vi "CR-导丝颗粒物检测3.vi"(8 "error in (no error)":errorcluster caption="错误输入（无错误）", 11 "名称或相对路径":string="Template Program") -> (0 "error in (no error) 2":errorcluster caption="错误输入（无错误）")   [LabVIEW 2017]
uses:
  Global System.vi
  <vilib>/Utility/xml.llb/Write to XML File(string).vi
  Picture/SaveButtom.ctl
panel:
  in  "获取图像":bool
  in  "ROI获取":bool
  in  "创建模板":bool
  in  "保存图像":bool
  out "添加的路径":path
  in  "刷新":bool
  in  "测试按钮":bool
  in  "保存按钮":bool
  in  "Main":enum32{"主参数", "模板匹配参数 ", "测试效果"}(tab)
  in  "导丝颗粒物检测3基础参数":T1={"IsNorImage"=TRUE, "Exposure Values"=100289, "ImagePath"=path "C:/Users/hedongpo/Desktop/514-hdp/Alignment Assemble System/Test Picture/B/3.bmp"} caption="参数界面" {"Exposure Values" scale=0.0..200000.0}
  in  "导丝颗粒物检测3参数":T3={"Rectangle"={"Left"=0, "Top"=0, "Right"=0, "Bottom"=0, "Rotation"=0.0}, "Threshold Limits (Threshold 1)"={"Lower value"=6.0, "Upper value"=245.0}, "Keep/Remove Particles "=FALSE, "Connectivity 4/8 (8) "=TRUE, "Selection Values (Particle Filter 1)"=[{"Measurement Parameter"=35, "Range Lower Value"=80.0, "Range Upper Value"=16332.0, "Range"=FALSE, "Measurement Type"=FALSE}], "Corner Options (Feature Detection 1)"={"Detector type"=enum."Harris Corner", "Kernel size"=7, "Min Corner Point Strength"=32.0}, "Pyramid level (Feature Detection 1)"=3, "Method "=2, "Look For"=0, "Method 2"=2, "ROI Descriptor (Clamp (Rake) 1)"={"Global Rectangle"=[162, 394, 420, 1807], "Contours"=[{"ID"=enum."External", "Type"=12, "Coordinates"=[162, 394, 420, 1807, 0]}]}} {"Method" items=["clustering", "entropy", "metric", "moments", "inter-class variance"]; "Look For" items=["Bright Objects", "Dark Objects"]; "Method 2" items=["clustering", "entropy", "metric", "moments", "inter-class variance"]; "ROI Descriptor (Clamp (Rake) 1)"."Contours"."Type" items=["No Selection", "Point", "Line", "Rectangle", "Oval", "Polygon", "Freehand Region", "Annulus", "Unused2", "Unused3", "Broken Line", "Freehand Line", "Rotated Rectangle"]; "Selection Values (Particle Filter 1)"."Measurement Parameter" items=["Center of Mass X", "Center of Mass Y", "First Pixel X", "First Pixel Y", "Bounding Rect Left", "Bounding Rect Top", "Bounding Rect Right", "Bounding Rect Bottom", "Max Feret Diameter Start X", "Max Feret Diameter Start Y", "Max Feret Diameter End X", "Max Feret Diameter End Y", "Max Horiz. Segment Length Left", "Max Horiz. Segment Length Right", "Max Horiz. Segment Length Row", "-", "Bounding Rect Width", "Bounding Rect Height", "Bounding Rect Diagonal", "Perimeter", "Convex Hull Perimeter", "Holes' Perimeter", "Max Feret Diameter", "Equivalent Ellipse Major Axis", "Equivalent Ellipse Minor Axis", "Equivalent Ellipse Minor Axis (Feret)", "Equivalent Rect Long Side", "Equivalent Rect Short Side", "Equivalent Rect Diagonal", "Equivalent Rect Short Side (Feret)", "Average Horiz. Segment Length", "Average Vert. Segment Length", "Hydraulic Radius", "Waddel Disk Diameter", "-", "Area", "Holes' Area", "Particle & Holes' Area", "Convex Hull Area", "Image Area", "-", "Number of Holes", "Number of Horiz. Segments", "Number of Vert. Segments", "-", "Orientation", "Max Feret Diameter Orientation", "-", "% Area/Image Area", "% Area/(Particle & Holes' Area)", "Ratio of Equivalent Ellipse Axes", "Ratio of Equivalent Rect Sides", "-", "Elongation Factor", "Compactness Factor", "Heywood Circularity Factor", "Type Factor", "-", "Sum X", "Sum Y", "Sum XX", "Sum XY", "Sum YY", "Sum XXX", "Sum XXY", "Sum XYY", "Sum YYY", "-", "Moment of Inertia XX", "Moment of Inertia XY", "Moment of Inertia YY", "Moment of Inertia XXX", "Moment of Inertia XXY", "Moment of Inertia XYY", "Moment of Inertia YYY", "Norm. Moment of Inertia XX", "Norm. Moment of Inertia XY", "Norm. Moment of Inertia YY", "Norm. Moment of Inertia XXX", "Norm. Moment of Inertia XXY", "Norm. Moment of Inertia XYY", "Norm. Moment of Inertia YYY", "Hu Moment 1", "Hu Moment 2", "Hu Moment 3", "Hu Moment 4", "Hu Moment 5", "Hu Moment 6", "Hu Moment 7"]; "Rectangle"."Rotation" min=-90.0 max=90.0 step=1.0 format="%.2f"; "Rectangle"."Left" scale=0.0..1024.0; "Rectangle"."Right" scale=0.0..1024.0}
  out "颗粒物有无显示":bool
  out "Number of Features Found":i32
  in  "颗粒物个数阈值":i32
  in  "Feature Points Strength":string[][](table)
  out "原始图像":T4(plugin-control)
  out "路径输出":path
  in  "Vision Paramter Save Buttom":T5
  out "system time":string
  in  "取消按钮":bool
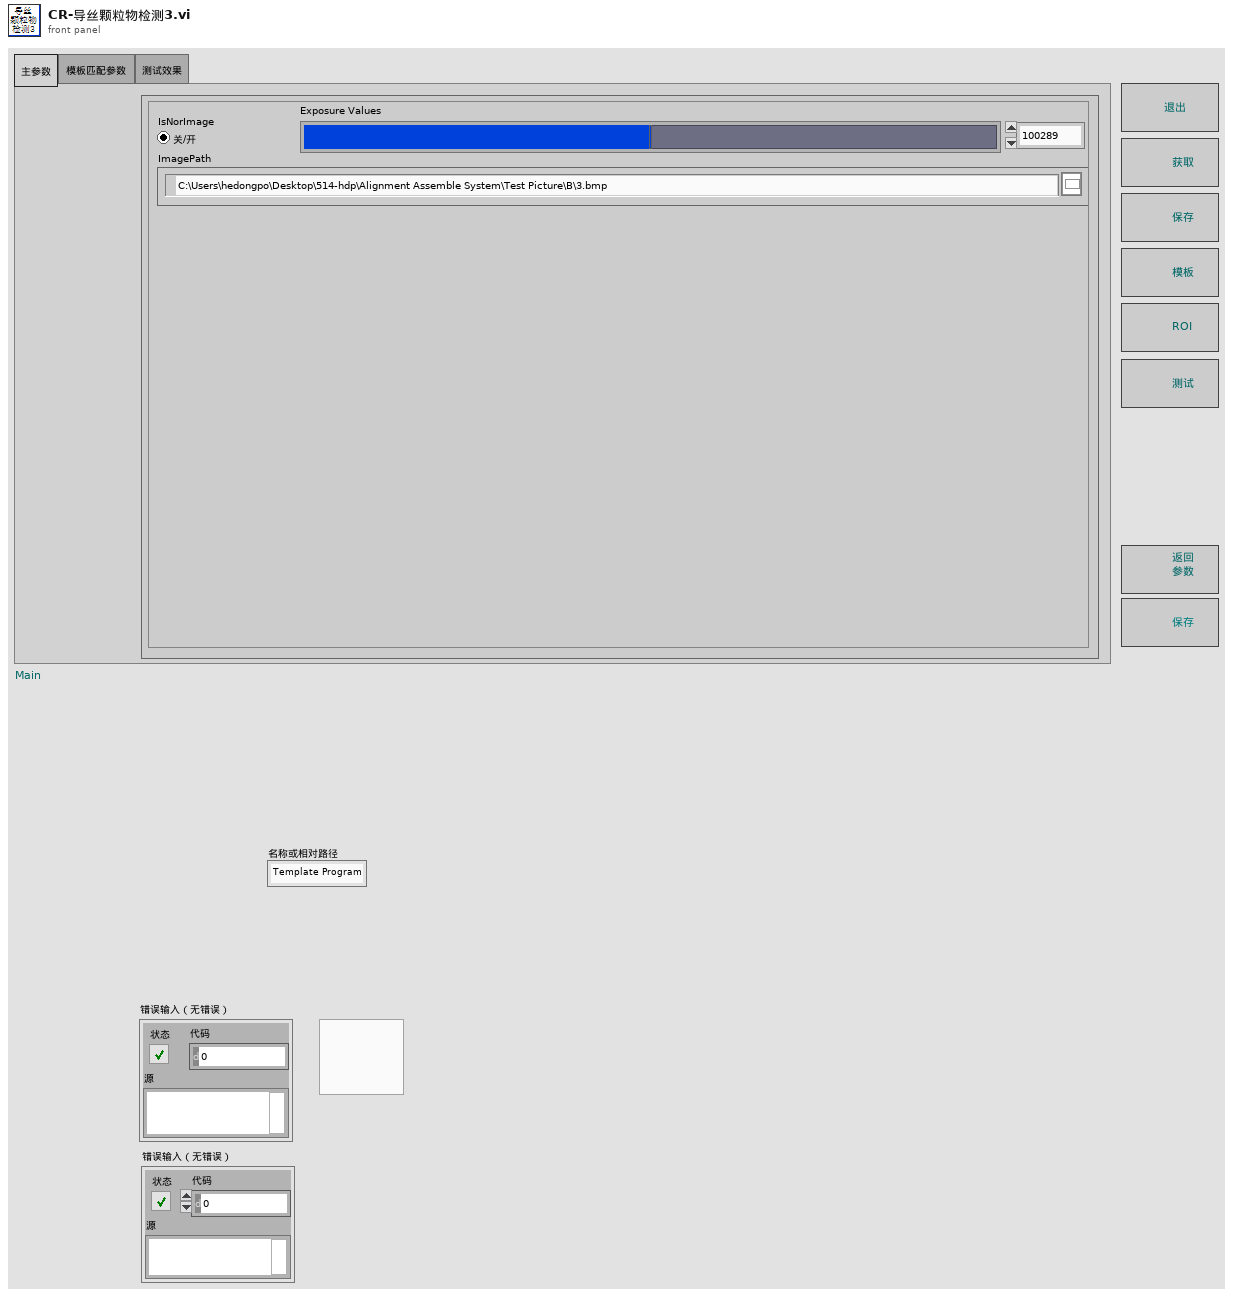
[diagram p1: front panel]
types:
  T1 = cluster{"IsNorImage":bool, "Exposure Values":u32, "ImagePath":path}
  T2 = typedef "IMAQ Rectangle" = cluster{"Left":i32, "Top":i32, "Right":i32, "Bottom":i32, "Rotation":dbl}
  T3 = cluster{"Rectangle":T2, "Threshold Limits (Threshold 1)":cluster{"Lower value":sgl, "Upper value":sgl}, "Keep/Remove Particles ":bool, "Connectivity 4/8 (8) ":bool, "Selection Values (Particle Filter 1)":cluster{"Measurement Parameter":i32, "Range Lower Value":dbl, "Range Upper Value":dbl, "Range":bool, "Measurement Type":bool}[], "Corner Options (Feature Detection 1)":cluster{"Detector type":enum32{"Harris Corner", "Shi-Tomasi Corner"}, "Kernel size":i32, "Min Corner Point Strength":dbl}, "Pyramid level (Feature Detection 1)":u32, "Method ":i32, "Look For":u32, "Method 2":i32, "ROI Descriptor (Clamp (Rake) 1)":cluster{"Global Rectangle":i32[], "Contours":cluster{"ID":enum32{"External", "Internal"}, "Type":u32, "Coordinates":i32[]}[]}}
  T4 = typedef "IMAQ Image.ctl" = refnum<image>
  T5 = typedef "SaveButtom.ctl" = bool
  T6 = cluster{"index":i32, "this vi":refnum<vi>, "error out":errorcluster}
  T7 = cluster{"master data":string, "priority":u16, "secondary data":string[]}
  T8 = cluster{"case name":string[], "queue array":refnum<queue>[]}
  T9 = cluster{"Global Rectangle":i32[], "Contours":cluster{"Contour Type":u32, "ROI Type":u32, "Points":i32[]}[]}
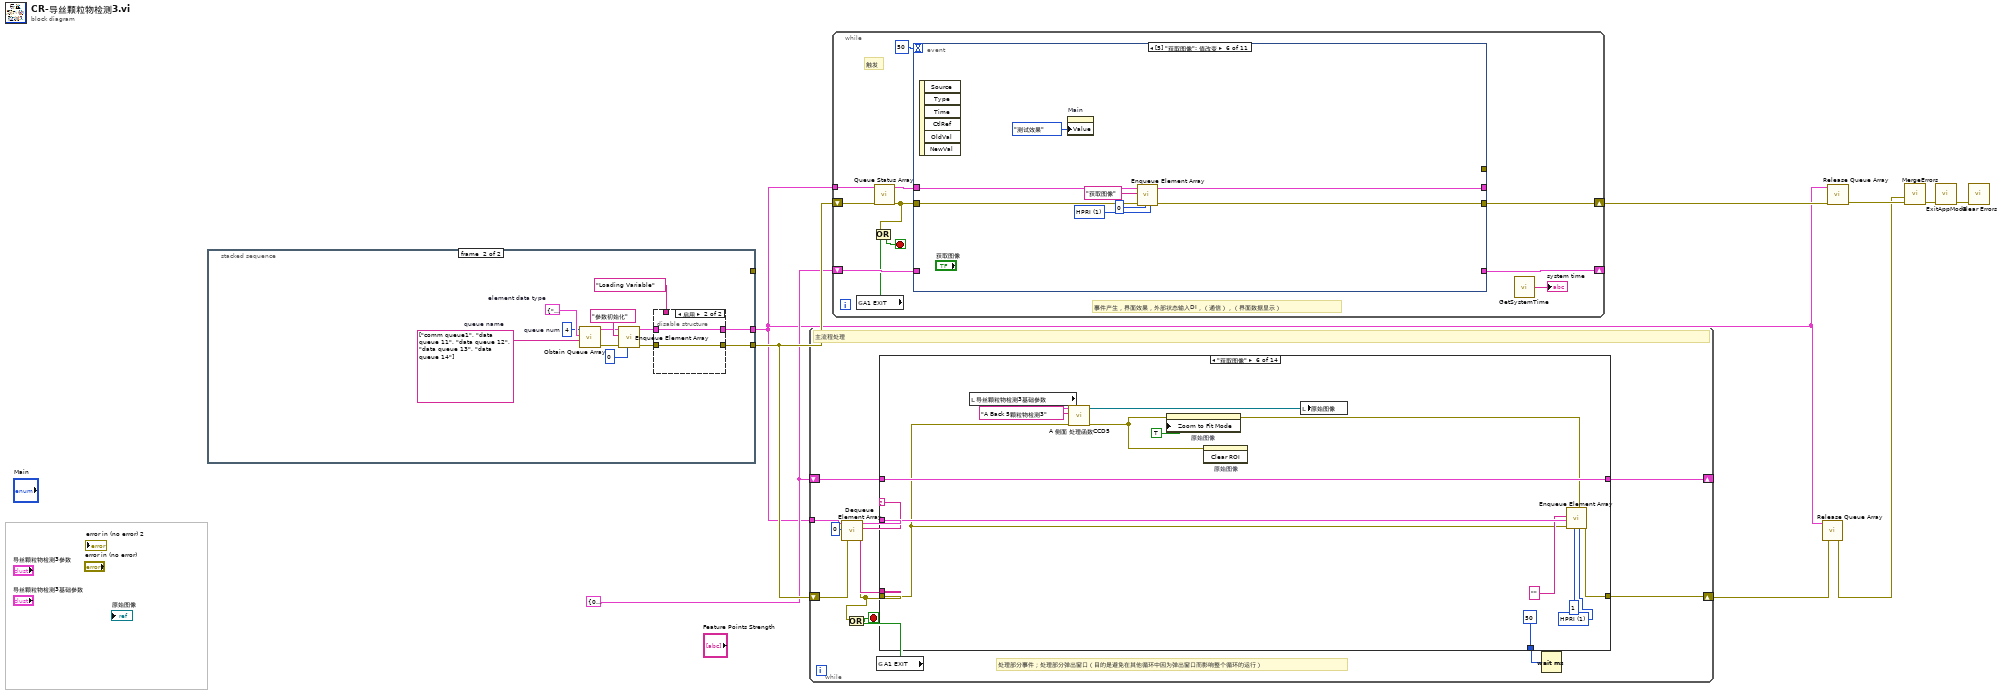
[diagram p0: block diagram]
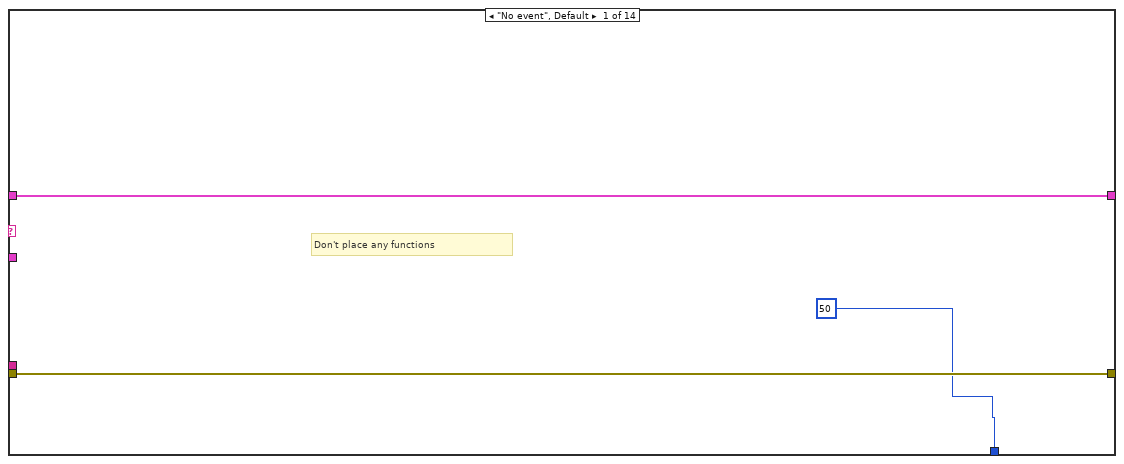
[diagram p2: hidden frame]
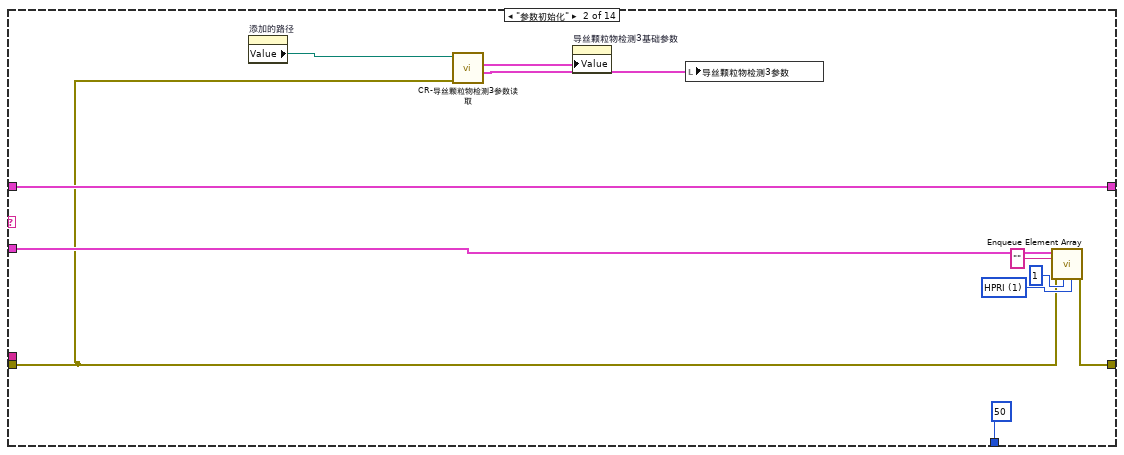
[diagram p3: hidden frame]
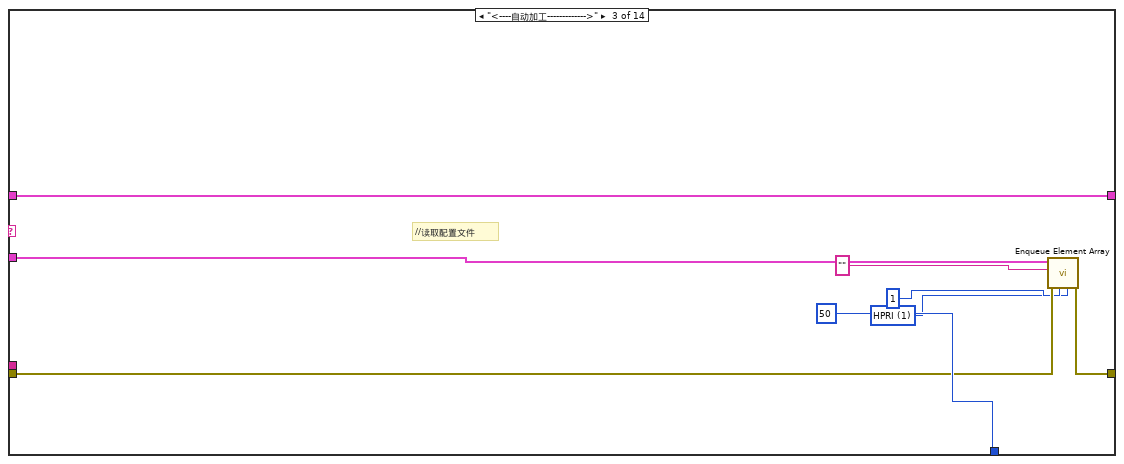
[diagram p4: hidden frame]
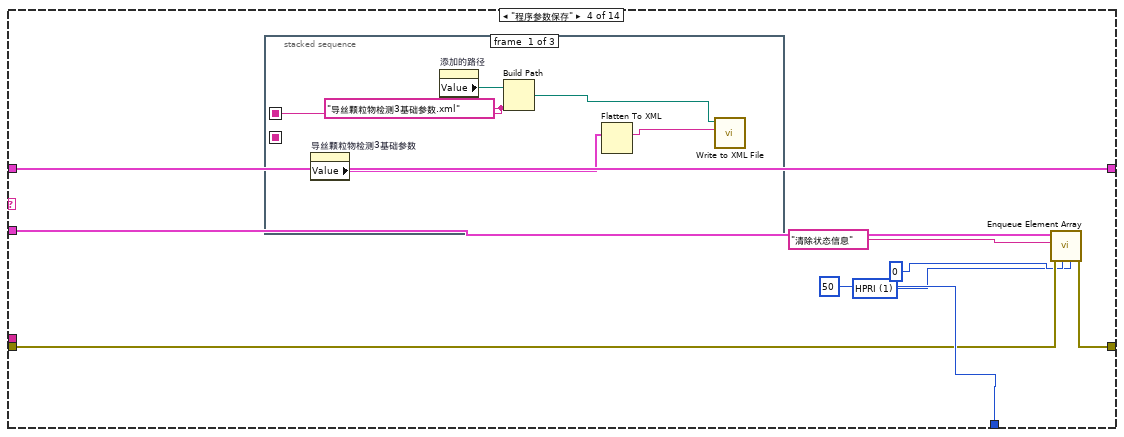
[diagram p5: hidden frame]
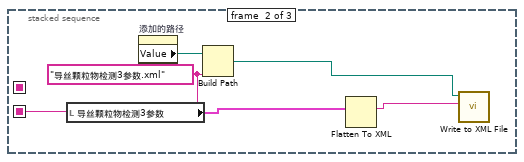
[diagram p6: hidden frame]
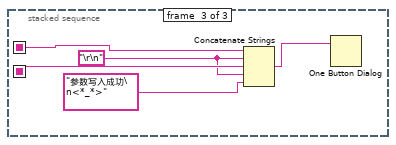
[diagram p7: hidden frame]
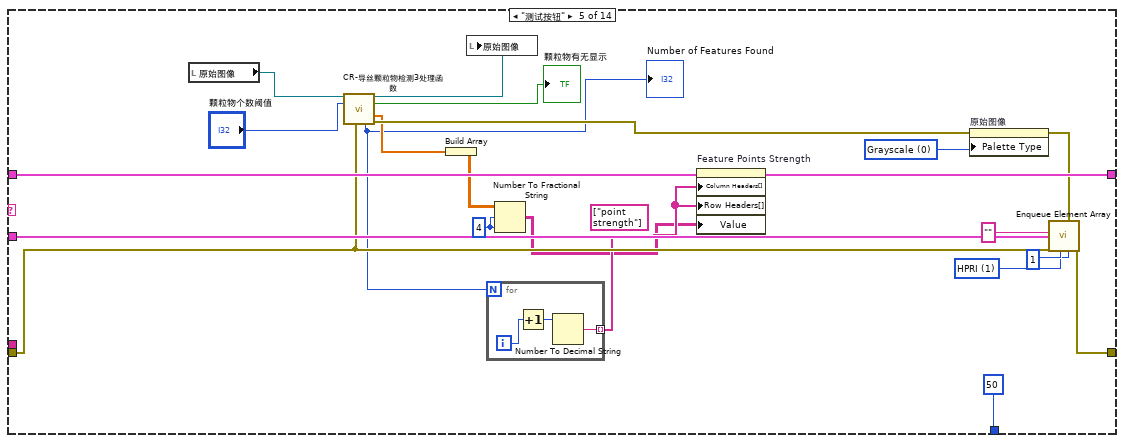
[diagram p8: hidden frame]
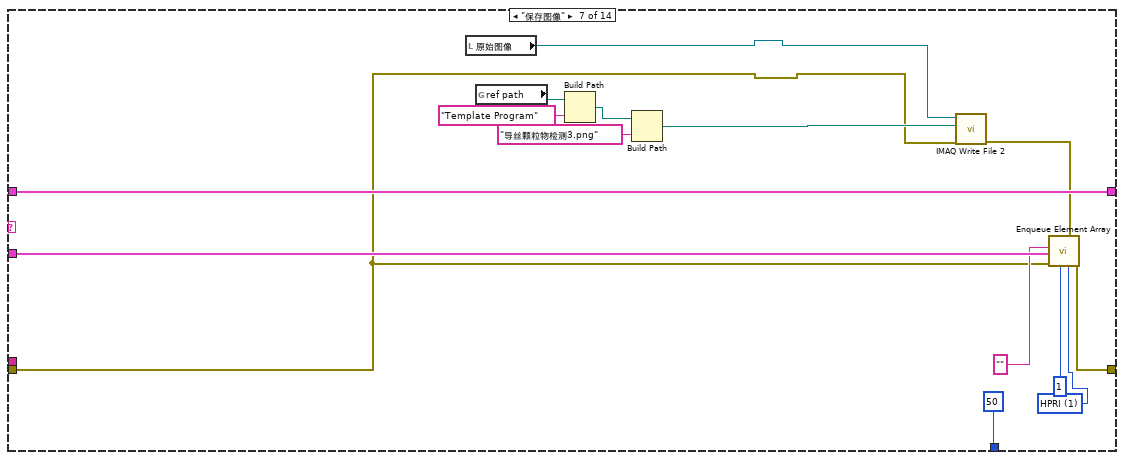
[diagram p9: hidden frame]
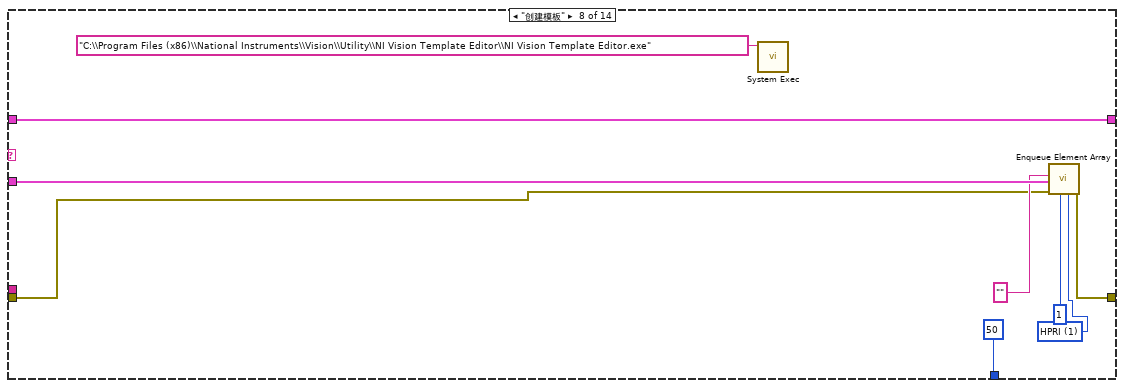
[diagram p10: hidden frame]
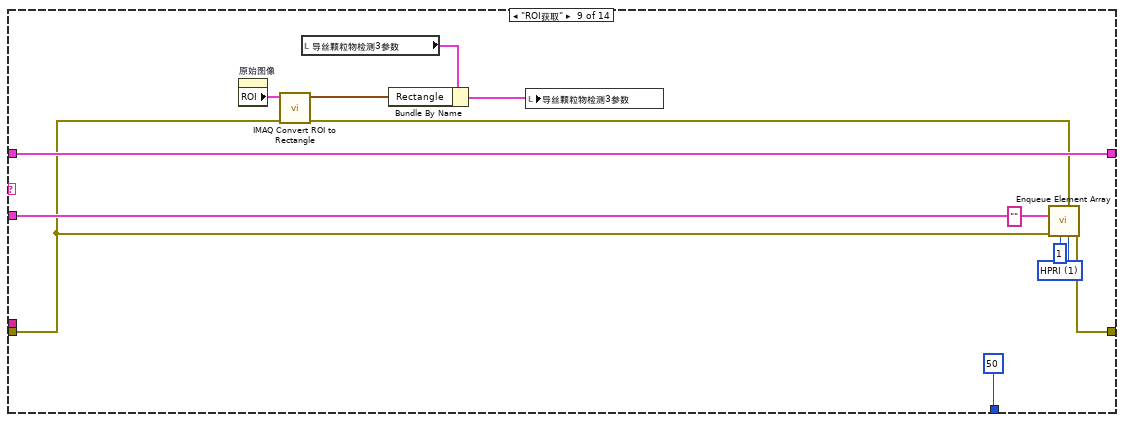
[diagram p11: hidden frame]
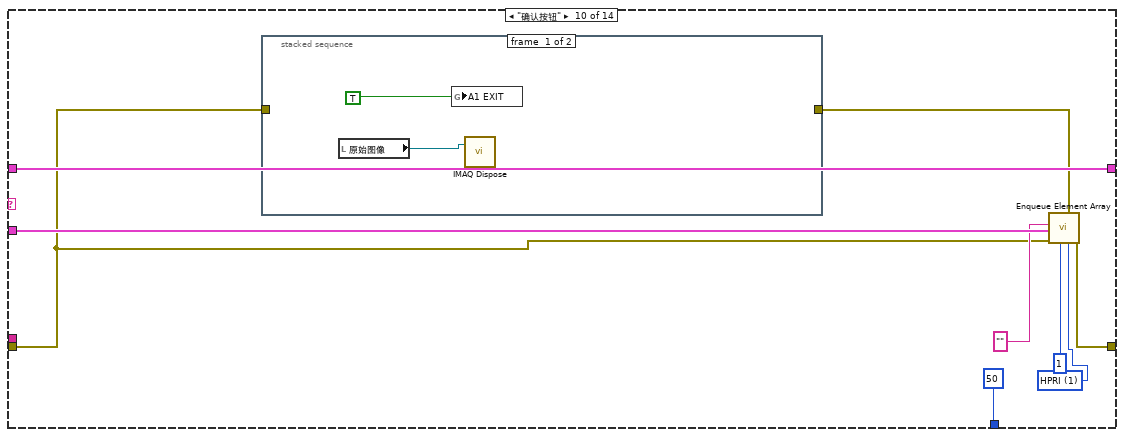
[diagram p12: hidden frame]
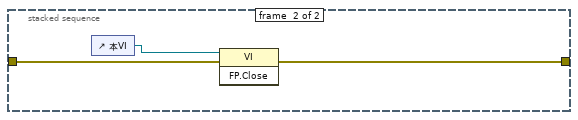
[diagram p13: hidden frame]
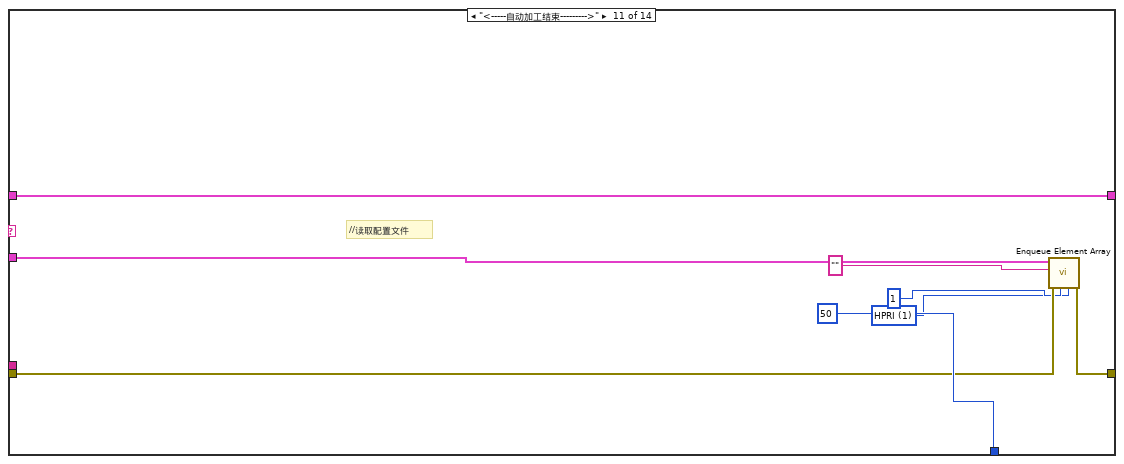
[diagram p14: hidden frame]
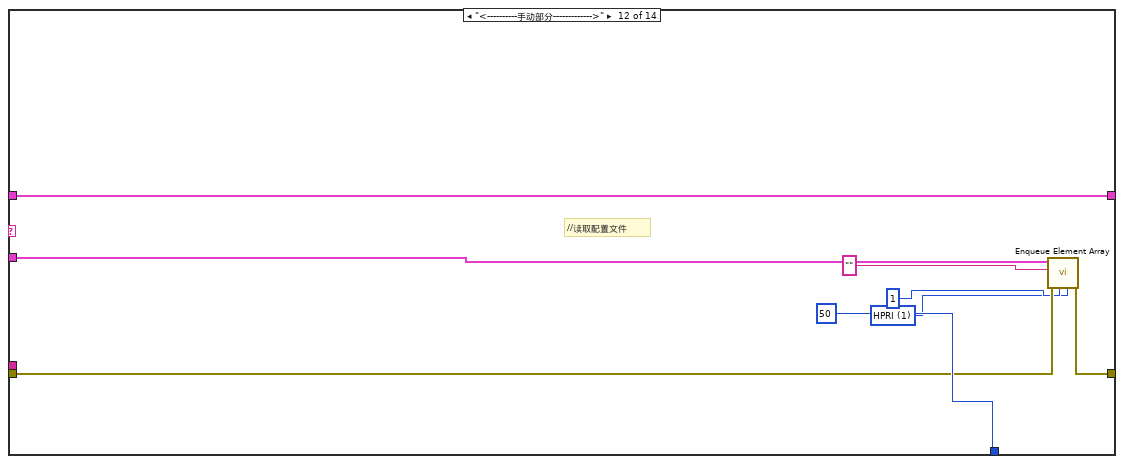
[diagram p15: hidden frame]
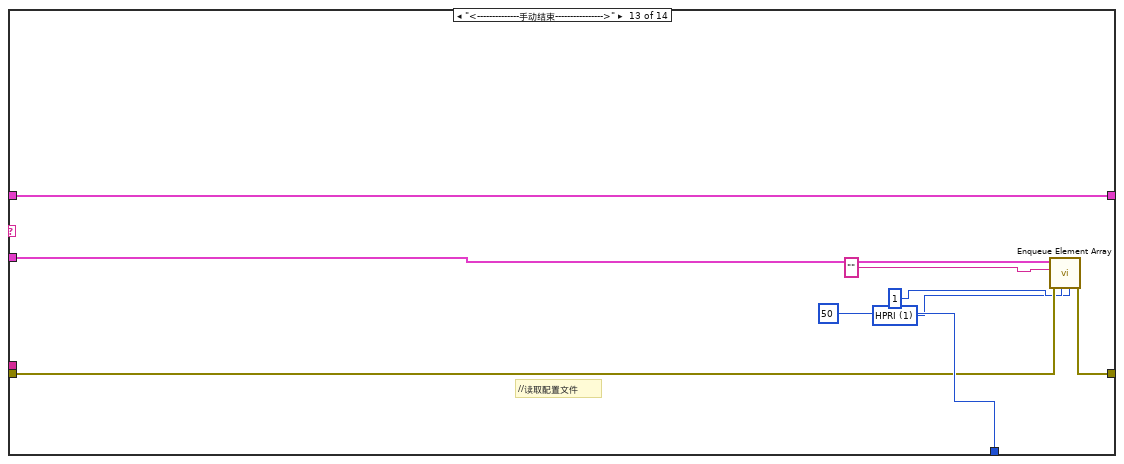
[diagram p16: hidden frame]
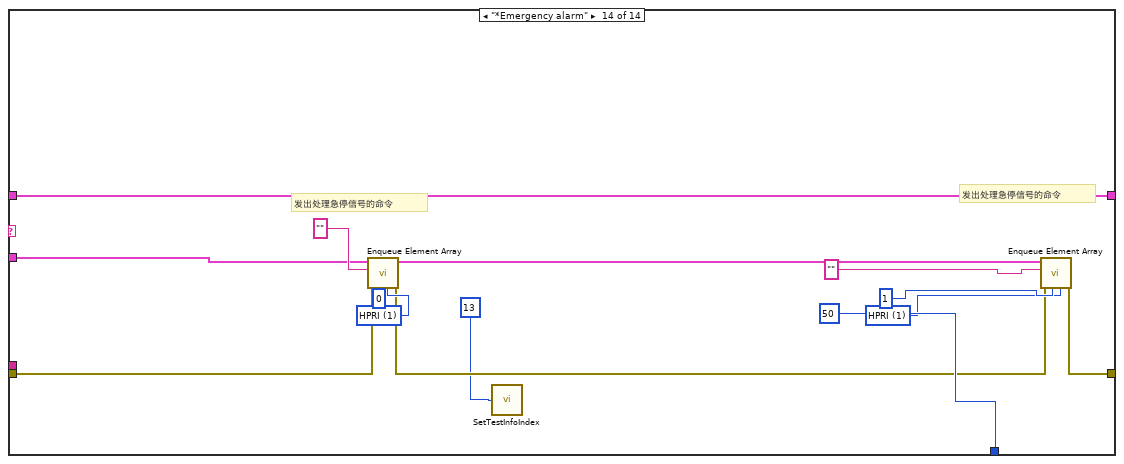
[diagram p17: hidden frame]
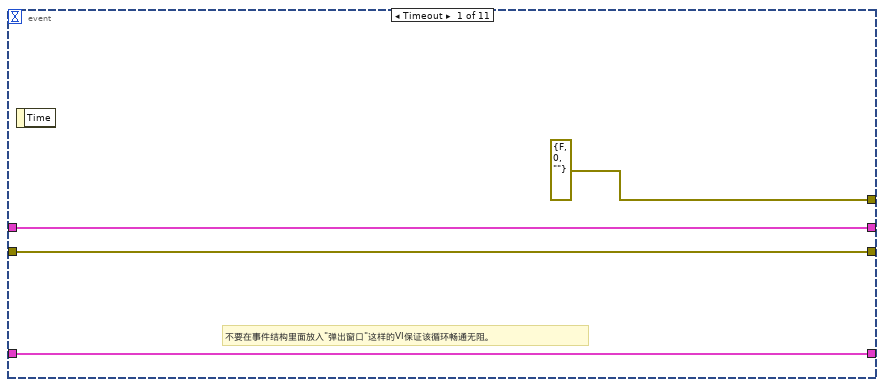
[diagram p18: hidden frame]
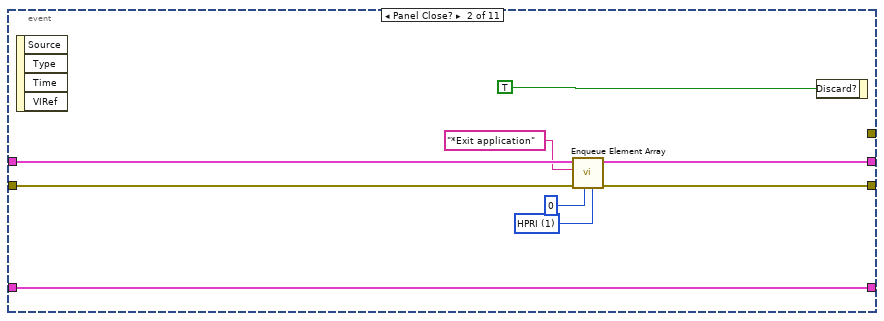
[diagram p19: hidden frame]
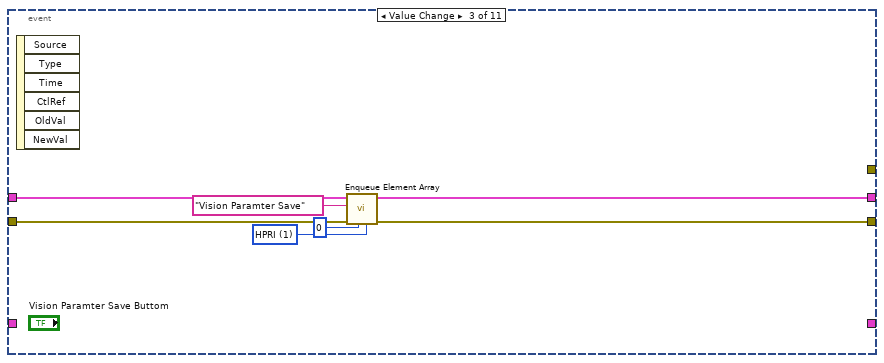
[diagram p20: hidden frame]
diagram:
  w4 = T6 {"index"=0, "this vi"=refnum, "error out"={"status"=FALSE, "code"=0, "source"=""}} ("parameter buffer")
  n1 = stacked-sequence {
    tunnel: [w15 _] -> _
    tunnel: [_ w19] -> w5
    tunnel: [_ w18] -> w1
    frame #0 {
      n2 = global read "Global System.vi" "ref path"() -> (w13:path)
      n3 = Build Path(base path=w13, name or relative path="Template Program" ("名称或相对路径")) -> (appended path=w11:path)
      n4 = property on="Main" class="TabCtl (严格)"("Value"=enum32{"主参数", "模板匹配参数 ", "测试效果"}."主参数" ("Main")) -> ()  [unwired: 2 in, 2 out]
      n5 = Build Path(base path=w11, name or relative path="名称或相对路径") -> (appended path=w17:path)
      "添加的路径" <- w17
      n6 = List Folder(path=w17) -> (path out=→"路径输出":path, error out=w15:errorcluster)  [unwired: 3 in, 2 out]
    }
    frame #1 {
      w27 = string[] ["comm queue1", "data queue 11", "data queue 12", "data queue 13", "data queue 14"]  # queue name
      w28 = 4  # queue num
      w29 = T7 {"master data"="", "priority"=0, "secondary data"=[]}  # element data type
      n7 = call "Obtain Queue Array.vi"("queue name"=w27, "element data type"=w29, "queue num"=w28) -> ("error out"=w23:errorcluster, "queue out"=w24:T8)  [unwired: 2 in, 1 out]
      n8 = call "Enqueue Element Array.vi"("queue index"=0, "error in"=w23, "master data"="参数初始化", "queue in"=w24) -> ("error out"=w22:errorcluster, "queue out"=w21:T8)  [unwired: 6 in]
      n9 = disable-structure shown="启用" {
        disable-tunnel: w22 -> [w35 w36]
        disable-tunnel: w21 -> [w34 w37]
        disable-tunnel: "Loading Variable" ("master data") -> [w33 _]
        disable-tunnel: [w31 w36] -> w19
        disable-tunnel: [w30 w37] -> w18
        frame Disabled {
          n10 = call "Enqueue Element Array.vi"("queue index"=12, "error in"=w35, "master data"=w33, "queue in"=w34) -> ("error out"=w31:errorcluster, "queue out"=w30:T8)  [unwired: 6 in]
        }
        frame Enabled {
        }
      }
    }
  }
  n11 = while {
    shift-right: [w50] -> w3
    shift-left: w5 -> [w41]
    shift-right: [w47] -> _
    shift-left: w4 -> [w48]
    tunnel: w1 -> [w43]
    stop <- w38 stop-if-true
    # "处理部分事件；处理部分弹出窗口（目的是避免在其他循环中因为弹出窗口而影响整个循环的运行）"
    # "主流程处理"
    n12 = call "Dequeue Element Array.vi"("queue in"=w43, "queue index"=0, "error in"=w41) -> ("queue out"=w46:T8, "master data"=w45:string, "secondary data"=w44:string[], "error out"=w40:errorcluster)  [unwired: 2 in, 1 out]
    n13 = global read "Global System.vi" "A1 EXIT"() -> (w39:bool)
    n14 = Or(x=w40, y=w39) -> (x .or. y?=w38:bool)
    n15 = case shown="\"获取图像\"" w45 {
      tunnel: w46 -> [_ w63 w71 w73 w115 w132 w147 w156 w169 w178 w191 w199 w207 w213]
      tunnel: w40 -> [w52 w56 w67 w77 w109 w123 w134 w150 w162 w172 w187 w195 w203 w210]
      tunnel: [w52 w62 w70 w79 w114 w131 w146 w155 w168 w177 w190 w198 w206 w221] -> w50
      tunnel: [50 50 50 50 50 50 50 50 50 50 50 50 50 50] -> w49
      tunnel: w48 -> [w53 w58 w68 w74 w110 w127 w142 w151 w164 w173 w188 w196 w204 w219]
      tunnel: [w53 w58 w68 w74 w110 w127 w142 w151 w164 w173 w188 w196 w204 w219] -> w47
      tunnel: w44 -> [_ _ _ _ _ _ _ _ _ _ _ _ _ _]
      frame "No event", Default {
        # "Don't place any functions"
      }
      frame "参数初始化" {
        w59 = u16 1 items=["HPRI"=1, "LPRI"=0] ("priority")
        n16 = property on="添加的路径" class="Path"() -> ("Value"=w57:path)  [unwired: 2 in, 2 out]
        n17 = call "CR-导丝颗粒物检测3参数读取.vi"("error in (no error)"=w56, "基路径"=w57) -> ("导丝颗粒物检测3参数"=w54:T3, "导丝颗粒物检测3基础参数"=w55:T1)  [unwired: 6 in, 1 out]
        n18 = property on="导丝颗粒物检测3基础参数" class="Clust (严格)"("Value"=w55) -> ()  [unwired: 2 in, 2 out]
        n19 = local write "导丝颗粒物检测3参数"(w54) -> ()
        n20 = call "Enqueue Element Array.vi"("priority"=w59, "queue index"=1, "error in"=w56, "master data"="" ("Element 1"), "queue in"=w63) -> ("error out"=w62:errorcluster)  [unwired: 5 in, 1 out]
      }
      frame "<----自动加工------------->" {
        w65 = u16 1 items=["HPRI"=1, "LPRI"=0] ("priority")
        # "//读取配置文件"
        n21 = call "Enqueue Element Array.vi"("priority"=w65, "queue index"=1, "error in"=w67, "master data"="" ("Element 1"), "queue in"=w71) -> ("error out"=w70:errorcluster)  [unwired: 5 in, 1 out]
      }
      frame "程序参数保存" {
        w75 = u16 1 items=["HPRI"=1, "LPRI"=0] ("priority")
        n22 = stacked-sequence {
          seq-local: [w81 _ _] -> [_ _ w94]
          seq-local: [_ w87 _] -> [_ _ w92]
          frame #0 {
            w81 = "导丝颗粒物检测3基础参数.xml" ("名称或相对路径")
            n23 = property on="导丝颗粒物检测3基础参数" class="Clust (严格)"() -> ("Value"=w84:T1)  [unwired: 2 in, 2 out]
            n24 = property on="添加的路径" class="Path"() -> ("Value"=w85:path)  [unwired: 2 in, 2 out]
            n25 = Build Path(base path=w85, name or relative path=w81) -> (appended path=w82:path)
            n26 = Flatten To XML(anything=w84) -> (xml string=w83:string)
            n27 = call-poly <vilib>:"Write to XML File.vi"("XML Input"=w83, "XML File Path"=w82) -> ()  [unwired: 7 in, 3 out]
          }
          frame #1 {
            w87 = "导丝颗粒物检测3参数.xml" ("名称或相对路径")
            n28 = local read "导丝颗粒物检测3参数"() -> (w86:T3)
            n29 = property on="添加的路径" class="Path"() -> ("Value"=w90:path)  [unwired: 2 in, 2 out]
            n30 = Build Path(base path=w90, name or relative path=w87) -> (appended path=w88:path)
            n31 = Flatten To XML(anything=w86) -> (xml string=w89:string)
            n32 = call-poly <vilib>:"Write to XML File.vi"("XML Input"=w89, "XML File Path"=w88) -> ()  [unwired: 7 in, 3 out]
          }
          frame #2 {
            w91 = "\r\n"
            n33 = Concatenate Strings(w94, w91, w92, w91, "参数写入成功\n<*_*>" ("消息")) -> (w93:string)
            n34 = One Button Dialog(message=w93) -> ()  [unwired: 1 in, 1 out]
          }
        }
        n35 = call "Enqueue Element Array.vi"("priority"=w75, "queue index"=0, "error in"=w77, "master data"="清除状态信息" ("Element 1"), "queue in"=w73) -> ("error out"=w79:errorcluster)  [unwired: 5 in, 1 out]
      }
      frame "测试按钮" {
        w102 = i16 4 ("精度(6)")
        (unwired) string[] ["point strength"] ("列首字符串[]")
        w106 = u32 0 items=["Grayscale", "Binary", "Gradient", "Rainbow", "Temperature", "User Defined", "Binary 16 Bit", "Gradient 16 Bit", "Rainbow 16 Bit", "Temperature 16 Bit", "User Defined 16 Bit"] ("Palette:Palette Type")
        w111 = u16 1 items=["HPRI"=1, "LPRI"=0] ("priority")
        n36 = local read "原始图像"() -> (w104:T4)
        n37 = call "CR-导丝颗粒物检测3处理函数.vi"("Image in"=w104, "颗粒物个数阈值"="颗粒物个数阈值", "error in (no error)"=w109) -> ("Image out"=w108:T4, "颗粒物有无显示"=→"颗粒物有无显示":bool, "颗粒物大小显示"=w100:dbl[], "Number of Features Found"=w98:i32, "error out"=w107:errorcluster)  [unwired: 7 in, 1 out]
        "Number of Features Found" <- w98
        n38 = Build Array(w100) -> (w101:dbl[][])
        n39 = local write "原始图像"(w108) -> ()
        n40 = for {
          N: w98 -> [_]
          tunnel: [w117] -> w97 mode=indexing
          i -> [w119]
          n41 = Increment(x=w119) -> (x+1=w118:i32)
          n42 = Number To Decimal String(number=w118) -> (decimal integer string=w117:string)  [unwired: 1 in]
        }
        n43 = Number To Fractional String(number=w101, width (-)=w102, precision (6)=w102) -> (F-format string=w96:string[][])  [unwired: 1 in]
        n44 = property on="Feature Points Strength" class="Tbl (严格)"("Column Headers[]"=w97, "Row Headers[]"=w97, "Value"=w96) -> ()  [unwired: 2 in, 2 out]
        n45 = property on="原始图像" class="ImageControl"(error in=w107, "Palette Type"=w106) -> (error out=w105:errorcluster)  [unwired: 1 in, 1 out]
        n46 = call "Enqueue Element Array.vi"("priority"=w111, "device error in"=w105, "queue index"=1, "error in"=w109, "master data"="" ("Element 1"), "queue in"=w115) -> ("error out"=w114:errorcluster)  [unwired: 4 in, 1 out]
      }
      frame "获取图像" {
        w128 = u16 1 items=["HPRI"=1, "LPRI"=0] ("priority")
        n47 = local read "导丝颗粒物检测3基础参数"() -> (w125:T1)
        n48 = call "A 侧面 处理函数CCD5.vi"("error in (no error)"=w123, "New Image"="A Back 5颗粒物检测3" ("Image Name"), "ParamsUI"=w125) -> ("error out"=w120:errorcluster, "Image out"=w124:T4)  [unwired: 5 in, 2 out]
        n49 = property on="原始图像" class="ImageControl"(error in=w120, "Zoom to Fit Mode"=TRUE) -> (error out=w121:errorcluster)  [unwired: 1 in, 1 out]
        n50 = invoke on="原始图像" class="ImageControl" method="Clear ROI"(error in=w120) -> ()  [unwired: 2 in, 3 out]
        n51 = local write "原始图像"(w124) -> ()
        n52 = call "Enqueue Element Array.vi"("priority"=w128, "device error in"=w121, "queue index"=1, "error in"=w123, "master data"="" ("Element 1"), "queue in"=w132) -> ("error out"=w131:errorcluster)  [unwired: 4 in, 1 out]
      }
      frame "保存图像" {
        w143 = u16 1 items=["HPRI"=1, "LPRI"=0] ("priority")
        n53 = local read "原始图像"() -> (w135:T4)
        n54 = global read "Global System.vi" "ref path"() -> (w141:path)
        n55 = Build Path(base path=w141, name or relative path="Template Program" ("名称或相对路径")) -> (appended path=w139:path)
        n56 = Build Path(base path=w139, name or relative path="导丝颗粒物检测3.png" ("名称或相对路径")) -> (appended path=w137:path)
        n57 = call-poly "IMAQ Write File 2"("error in (no error)"=w134, "File Path"=w137, "Image"=w135) -> ("error out"=w136:errorcluster)  [unwired: 7 in, 1 out]
        n58 = call "Enqueue Element Array.vi"("priority"=w143, "device error in"=w136, "queue index"=1, "error in"=w134, "master data"="" ("Element 1"), "queue in"=w147) -> ("error out"=w146:errorcluster)  [unwired: 4 in, 1 out]
      }
      frame "创建模板" {
        w152 = u16 1 items=["HPRI"=1, "LPRI"=0] ("priority")
        n59 = call <vilib>:"System Exec.vi"("command line"="C:\\Program Files (x86)\\National Instruments\\Vision\\Utility\\NI Vision Template Editor\\NI Vision Template Editor.exe") -> ()  [unwired: 7 in, 4 out]
        n60 = call "Enqueue Element Array.vi"("priority"=w152, "queue index"=1, "error in"=w150, "master data"="" ("Element 1"), "queue in"=w156) -> ("error out"=w155:errorcluster)  [unwired: 5 in, 1 out]
      }
      frame "ROI获取" {
        w165 = u16 1 items=["HPRI"=1, "LPRI"=0] ("priority")
        n61 = property on="原始图像" class="ImageControl"() -> ("ROI"=w163:T9)  [unwired: 2 in, 2 out]
        n62 = call "IMAQ Convert ROI to Rectangle"("error in (no error)"=w162, "ROI Descriptor"=w163) -> ("error out"=w158:errorcluster, "Rectangle"=w160:T2)  [unwired: 7 in]
        n63 = local read "导丝颗粒物检测3参数"() -> (w161:T3)
        n64 = Bundle By Name(cluster=w161, "Rectangle"=w160) -> (w159:T3)
        n65 = local write "导丝颗粒物检测3参数"(w159) -> ()
        n66 = call "Enqueue Element Array.vi"("priority"=w165, "device error in"=w158, "queue index"=1, "error in"=w162, "master data"="" ("Element 1"), "queue in"=w169) -> ("error out"=w168:errorcluster)  [unwired: 4 in, 1 out]
      }
      frame "确认按钮" {
        w174 = u16 1 items=["HPRI"=1, "LPRI"=0] ("priority")
        n67 = stacked-sequence {
          tunnel: w172 -> [_ w183]
          tunnel: [_ w182] -> w171
          frame #0 {
            n68 = local read "原始图像"() -> (w180:T4)
            n69 = global write "Global System.vi" "A1 EXIT"(TRUE ("EXIT")) -> ()
            n70 = call "IMAQ Dispose"("Image"=w180) -> ()  [unwired: 5 in, 1 out]
          }
          frame #1 {
            n71 = control-ref of="本VI"() -> (w184:refnum<vi>)
            n72 = invoke class="VI" method="FP.Close"(reference=w184, error in=w183) -> (error out=w182:errorcluster)  [unwired: 1 in, 2 out]
          }
        }
        n73 = call "Enqueue Element Array.vi"("priority"=w174, "device error in"=w171, "queue index"=1, "error in"=w172, "master data"="" ("Element 1"), "queue in"=w178) -> ("error out"=w177:errorcluster)  [unwired: 4 in, 1 out]
      }
      frame "<-----自动加工结束--------->" {
        w185 = u16 1 items=["HPRI"=1, "LPRI"=0] ("priority")
        # "//读取配置文件"
        n74 = call "Enqueue Element Array.vi"("priority"=w185, "queue index"=1, "error in"=w187, "master data"="" ("Element 1"), "queue in"=w191) -> ("error out"=w190:errorcluster)  [unwired: 5 in, 1 out]
      }
      frame "<----------手动部分------------->" {
        w193 = u16 1 items=["HPRI"=1, "LPRI"=0] ("priority")
        # "//读取配置文件"
        n75 = call "Enqueue Element Array.vi"("priority"=w193, "queue index"=1, "error in"=w195, "master data"="" ("Element 1"), "queue in"=w199) -> ("error out"=w198:errorcluster)  [unwired: 5 in, 1 out]
      }
      frame "<--------------手动结束---------------->" {
        w201 = u16 1 items=["HPRI"=1, "LPRI"=0] ("priority")
        # "//读取配置文件"
        n76 = call "Enqueue Element Array.vi"("priority"=w201, "queue index"=1, "error in"=w203, "master data"="" ("Element 1"), "queue in"=w207) -> ("error out"=w206:errorcluster)  [unwired: 5 in, 1 out]
      }
      frame "*Emergency alarm" {
        w216 = u16 1 items=["HPRI"=1, "LPRI"=0] ("priority")
        w217 = u16 1 items=["HPRI"=1, "LPRI"=0] ("priority")
        # "发出处理急停信号的命令"
        # "发出处理急停信号的命令"
        n77 = call "Enqueue Element Array.vi"("priority"=w216, "queue index"=0, "error in"=w210, "master data"="" ("Element 1"), "queue in"=w213) -> ("error out"=w211:errorcluster, "queue out"=w212:T8)  [unwired: 5 in]
        n78 = call "SetTestInfoIndex.vi"("test info index"=13) -> ()
        n79 = call "Enqueue Element Array.vi"("priority"=w217, "queue index"=1, "error in"=w211, "master data"="" ("Element 1"), "queue in"=w212) -> ("error out"=w221:errorcluster)  [unwired: 5 in, 1 out]
      }
    }
    n80 = Wait (ms)(milliseconds to wait=w49) -> ()  [unwired: 1 out]
  }
  n81 = while {
    shift-right: [w226] -> w6
    shift-left: w5 -> [w230]
    shift-right: [w228] -> _
    shift-left: w4 -> [w229]
    tunnel: w1 -> [w232]
    stop <- w223 stop-if-true
    # "触发"
    # "事件产生，界面效果，外部状态输入DI，（通信），（界面数据显示）"
    n82 = global read "Global System.vi" "A1 EXIT"() -> (w224:bool)
    n83 = call "Queue Status Array.vi"("error in (no error)"=w230, "queue in"=w232) -> ("error out"=w225:errorcluster, "queue out"=w227:T8)  [unwired: 4 in]
    n84 = Or(x=w225, y=w224) -> (x .or. y?=w223:bool)
    n85 = event shown="[5] \"获取图像\": 值改变" {
      selector: _ -> [_ _ _ _ _ _ _ _ _ _ _]
      dyn-events: _ -> [_ _ _ _ _ _ _ _ _ _ _]
      timeout: 50 -> [_ _ _ _ _ _ _ _ _ _ _]
      tunnel: w229 -> [w237 w245 _ _ _ _ _ _ _ _ _]
      tunnel: [w237 w245 _ _ _ _ _ _ _ _ _] -> w228
      tunnel: [errorcluster {"status"=FALSE, "code"=0, "source"=""} ("error out") _ _ _ _ _ _ _ _ _ _] -> _
      tunnel: w227 -> [w235 w244 w250 w257 w264 w272 w279 w286 w294 w302 w310]
      tunnel: w225 -> [w234 w243 w249 w256 w263 w271 w278 w285 w293 w301 w309]
      tunnel: [w234 w242 w247 w254 w261 w269 w276 w283 w291 w299 w307] -> w226
      tunnel: [w235 w241 w248 w255 w262 w270 w277 w284 w292 w300 w308] -> _
      event Timeout {
        # "不要在事件结构里面放入\"弹出窗口\"这样的VI保证该循环畅通无阻。"
        n86 = event-data() -> ()  [unwired: 1 in, 1 out]
      }
      event Panel Close? {
        w239 = u16 1 items=["HPRI"=1, "LPRI"=0] ("priority")
        n87 = event-data() -> ()  [unwired: 1 in, 4 out]
        n88 = call "Enqueue Element Array.vi"("priority"=w239, "queue index"=0, "error in"=w243, "master data"="*Exit application", "queue in"=w244) -> ("error out"=w242:errorcluster, "queue out"=w241:T8)  [unwired: 5 in]
        n89 = event-data("Discard?"=TRUE) -> ()  [unwired: 1 in, 1 out]
      }
      event Value Change {
        w252 = u16 1 items=["HPRI"=1, "LPRI"=0] ("priority")
        n90 = event-data() -> ()  [unwired: 1 in, 6 out]
        n91 = call "Enqueue Element Array.vi"("priority"=w252, "queue index"=0, "error in"=w249, "master data"="Vision Paramter Save", "queue in"=w250) -> ("error out"=w247:errorcluster, "queue out"=w248:T8)  [unwired: 5 in]
      }
      event "取消按钮": Value Change {
        w259 = u16 1 items=["HPRI"=1, "LPRI"=0] ("priority")
        n92 = event-data() -> ()  [unwired: 1 in, 6 out]
        n93 = call "Enqueue Element Array.vi"("priority"=w259, "queue index"=0, "error in"=w256, "master data"="确认按钮", "queue in"=w257) -> ("error out"=w254:errorcluster, "queue out"=w255:T8)  [unwired: 5 in]
      }
      event "保存按钮": Value Change {
        w266 = u16 1 items=["HPRI"=1, "LPRI"=0] ("priority")
        n94 = event-data() -> ()  [unwired: 1 in, 6 out]
        n95 = call "Enqueue Element Array.vi"("priority"=w266, "queue index"=0, "error in"=w263, "master data"="程序参数保存", "queue in"=w264) -> ("error out"=w261:errorcluster, "queue out"=w262:T8)  [unwired: 5 in]
      }
      event "获取图像": Value Change {
        w274 = u16 1 items=["HPRI"=1, "LPRI"=0] ("priority")
        n96 = event-data() -> ()  [unwired: 1 in, 6 out]
        n97 = property on="Main" class="TabCtl (严格)"("Value"=enum32{"主参数", "模板匹配参数 ", "测试效果"}."测试效果" ("Main")) -> ()  [unwired: 2 in, 2 out]
        n98 = call "Enqueue Element Array.vi"("priority"=w274, "queue index"=0, "error in"=w271, "master data"="获取图像", "queue in"=w272) -> ("error out"=w269:errorcluster, "queue out"=w270:T8)  [unwired: 5 in]
      }
      event "保存图像": Value Change {
        w281 = u16 1 items=["HPRI"=1, "LPRI"=0] ("priority")
        n99 = event-data() -> ()  [unwired: 1 in, 6 out]
        n100 = call "Enqueue Element Array.vi"("priority"=w281, "queue index"=0, "error in"=w278, "master data"="保存图像", "queue in"=w279) -> ("error out"=w276:errorcluster, "queue out"=w277:T8)  [unwired: 5 in]
      }
      event "创建模板": Value Change {
        w288 = u16 1 items=["HPRI"=1, "LPRI"=0] ("priority")
        n101 = event-data() -> ()  [unwired: 1 in, 6 out]
        n102 = call "Enqueue Element Array.vi"("priority"=w288, "queue index"=0, "error in"=w285, "master data"="创建模板", "queue in"=w286) -> ("error out"=w283:errorcluster, "queue out"=w284:T8)  [unwired: 5 in]
      }
      event "ROI获取": Value Change {
        w296 = u16 1 items=["HPRI"=1, "LPRI"=0] ("priority")
        n103 = event-data() -> ()  [unwired: 1 in, 6 out]
        n104 = property on="Main" class="TabCtl (严格)"("Value"=enum32{"主参数", "模板匹配参数 ", "测试效果"}."模板匹配参数 " ("Main")) -> ()  [unwired: 2 in, 2 out]
        n105 = call "Enqueue Element Array.vi"("priority"=w296, "queue index"=0, "error in"=w293, "master data"="ROI获取", "queue in"=w294) -> ("error out"=w291:errorcluster, "queue out"=w292:T8)  [unwired: 5 in]
      }
      event "测试按钮": Value Change {
        w304 = u16 1 items=["HPRI"=1, "LPRI"=0] ("priority")
        n106 = event-data() -> ()  [unwired: 1 in, 6 out]
        n107 = property on="Main" class="TabCtl (严格)"("Value"=enum32{"主参数", "模板匹配参数 ", "测试效果"}."测试效果" ("Main")) -> ()  [unwired: 2 in, 2 out]
        n108 = call "Enqueue Element Array.vi"("priority"=w304, "queue index"=0, "error in"=w301, "master data"="测试按钮", "queue in"=w302) -> ("error out"=w299:errorcluster, "queue out"=w300:T8)  [unwired: 5 in]
      }
      event "刷新": Value Change {
        n109 = event-data() -> ()  [unwired: 1 in, 6 out]
        n110 = disable-structure shown="禁用" {
          disable-tunnel: w310 -> [w314 _]
          disable-tunnel: w309 -> [w313 _]
          disable-tunnel: [w312 _] -> w308
          disable-tunnel: [w311 _] -> w307
          frame Disabled {
            w316 = u16 1 items=["HPRI"=1, "LPRI"=0] ("priority")
            # "刷新"
            n111 = call "Enqueue Element Array.vi"("priority"=w316, "queue index"=0, "error in"=w313, "master data"="刷新", "queue in"=w314) -> ("error out"=w311:errorcluster, "queue out"=w312:T8)  [unwired: 5 in]
          }
          frame Enabled {
          }
        }
        n112 = property on="Main" class="TabCtl (严格)"("Value"=enum32{"主参数", "模板匹配参数 ", "测试效果"}."模板匹配参数 " ("Main")) -> ()  [unwired: 2 in, 2 out]
      }
    }
    n113 = call "GetSystemTime.vi"() -> ("date/time string"=→"system time":string)  [unwired: 7 in]
  }
  n114 = call "Release Queue Array.vi"("error in"=w3, "queue in"=w1) -> ("error out"=w2:errorcluster)  [unwired: 2 in, 3 out]
  n115 = call "Release Queue Array.vi"("error in"=w6, "queue in"=w1) -> ("error out"=w9:errorcluster)  [unwired: 2 in, 3 out]
  n116 = call "MergeErrors.vi"("error in 3 (no error)"=w2, "error in 4 (no error)"=w9) -> ("error out"=w8:errorcluster)  [unwired: 6 in]
  n117 = call "ExitAppMode.vi"("error in (no error)"=w8) -> ("error out"=w7:errorcluster)  [unwired: 10 in]
  n118 = call <vilib>:"Clear Errors.vi"("error in (no error)"=w7) -> ()  [unwired: 5 in, 2 out]
